vi "Read Fuel.vi"(8 "error in":errorcluster, 11 "Serial sessions":refnum<class "MB_Master_Serial.lvclass">[](array[class])) -> (0 "error out":errorcluster, 2 "Serial out":refnum<class "MB_Master_Serial.lvclass">[](array[class]), 3 "Fuel Flows":dbl[][](array[numeric]))   [LabVIEW 2017, in "Akwizycja.lvlib"]
uses:
  Akwizycja.lvlib
  <vilib>/Plasmionique/MB Master/MB_Master_Serial/MB_Master_Serial.lvclass
  D:/Program Files (x86)/National Instruments/LabVIEW 2017/vi.lib/Plasmionique/MB Master/MB_Master/MB_Master.lvclass
  <vilib>/Plasmionique/MB Master/MB Master.lvlib
  <vilib>/Utility/config.llb/NI_LVConfig.lvlib
panel:
  in  "P_Rx":T1
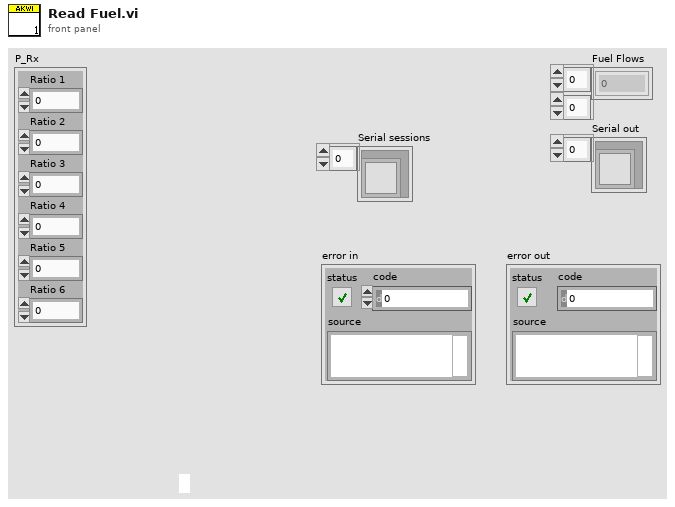
[diagram p1: front panel]
types:
  T1 = cluster{"Ratio 1":dbl, "Ratio 2":dbl, "Ratio 3":dbl, "Ratio 4":dbl, "Ratio 5":dbl, "Ratio 6":dbl}
  T2 = typedef "NI_LVConfig.lvlib/Config Data RefNum.ctl" = refnum<k1>
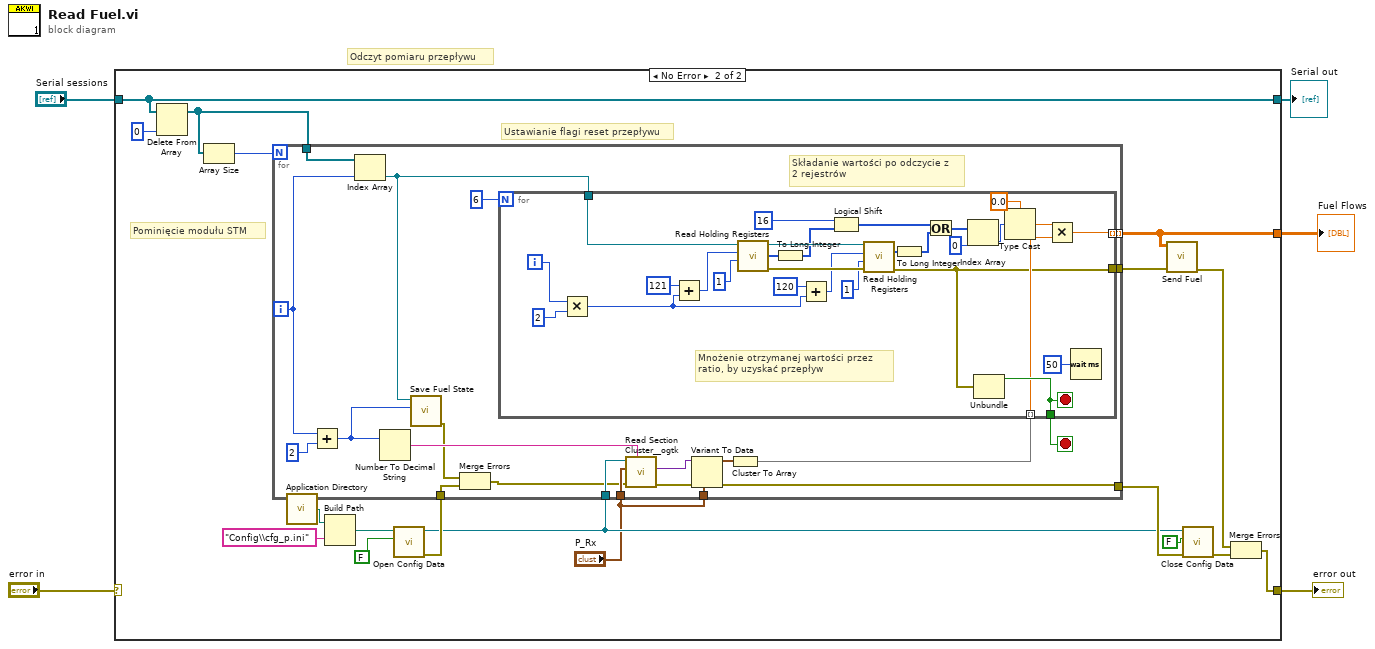
[diagram p0: block diagram]
diagram:
  # "Odczyt pomiaru przepływu"
  n1 = case shown="No Error" "error in" {
    selector: "error in" -> [w7 _]
    tunnel: "Serial sessions" -> [w6 w8]
    tunnel: [w7 w19] -> w4
    tunnel: [_ w10] -> w2
    tunnel: [w6 w8] -> w1
    frame Error {
    }
    frame No Error {
      # "Pominięcie modułu STM"
      # "Ustawianie flagi reset przepływu"
      n2 = Delete From Array(array=w8, index=0) -> (array with subset deleted=w9:refnum<class "MB_Master_Serial.lvclass">[])  [unwired: 1 in, 1 out]
      n3 = Array Size(array=w9) -> (size(s)=w16:i32)
      n4 = call <vilib>:"Application Directory.vi"() -> ("Application Directory"=w20:path)
      n5 = Build Path(base path=w20, name or relative path="Config\\cfg_p.ini") -> (appended path=w22:path)
      n6 = call <vilib>:"Open Config Data.vi"("create file if necessary (T)"=FALSE, "configuration file path"=w22) -> ("error out"=w18:errorcluster, "refnum"=w14:T2)  [unwired: 7 in, 1 out]
      n7 = for {
        N: w16 -> [_]
        tunnel: [w32] -> w25
        tunnel: w9 -> [w43]
        tunnel: [w45] -> w12
        tunnel: w18 -> [w28]
        tunnel: [w40] -> w10 mode=indexing
        tunnel: w14 -> [w39]
        tunnel: "P_Rx" -> [w38]
        tunnel: "P_Rx" -> [w35]
        i -> [w42]
        stop <- w44 stop-if-true
        # "Składanie wartości po odczycie z\n2 rejestrów"
        n8 = Add(x=w42, y=2) -> (x+y=w30:i32)
        n9 = Index Array(array=w43, index=w42) -> (element=w29:refnum<class "MB_Master_Serial.lvclass">)
        n10 = Number To Decimal String(number=w30) -> (decimal integer string=w37:string)  [unwired: 1 in]
        n11 = call "Save Fuel State.vi"("Slave ID"=w30, "Session in"=w29) -> ("error out"=w26:errorcluster)  [unwired: 9 in]
        n12 = Merge Errors(w26, w28) -> (w27:errorcluster)
        n13 = call <userlib>:"Read Section Cluster__ogtk.vi"("section (optional)"=w37, "error in (no error)"=w27, "Section Formatted Cluster Type"=w38, "refnum"=w39) -> ("error out"=w36:errorcluster, "Section Formatted Cluster"=w34:variant)  [unwired: 3 in, 3 out]
        n14 = Variant To Data(error in=w36, type=w35, Variant=w34) -> (data=w33:T1, error out=w32:errorcluster)
        n15 = Cluster To Array(cluster=w33) -> (array=w31:dbl[])
        n16 = for {
          N: 6 ("Numeric Control") -> [_]
          tunnel: w29 -> [w47]
          tunnel: [w48] -> w45
          tunnel: [w74] -> w44
          tunnel: [w55] -> w40 mode=indexing
          tunnel: w31 -> [w61] mode=indexing
          i -> [w66]
          stop <- w74 stop-if-true
          # "Mnożenie otrzymanej wartości przez \nratio, by uzyskać przepływ"
          n17 = Multiply(x=w66, y=2) -> (x*y=w64:i32)
          n18 = Add(x=u16 121 ("starting address"), y=w64) -> (x+y=w72:i32)
          n19 = call <vilib>:"Read Holding Registers.vi"("quantity"=u16 1, "starting address"=w72, "MB session in"=w47) -> ("error out"=w68:errorcluster, "Registers"=w54:u16[], "MB session out"=w69:refnum<class "MB_Master_Serial.lvclass">)  [unwired: 6 in]
          n20 = To Long Integer(number=w54) -> (32bit integer=w53:i32[])
          n21 = Add(x=u16 120 ("starting address"), y=w64) -> (x+y=w63:i32)
          n22 = Logical Shift(y=16, x=w53) -> (x << y=w58:i32[])
          n23 = call <vilib>:"Read Holding Registers.vi"("error in (no error)"=w68, "quantity"=u16 1, "starting address"=w63, "MB session in"=w69) -> ("error out"=w48:errorcluster, "Registers"=w59:u16[])  [unwired: 5 in, 1 out]
          n24 = To Long Integer(number=w59) -> (32bit integer=w60:i32[])
          n25 = Or(x=w58, y=w60) -> (x .or. y?=w57:i32[])
          n26 = Index Array(array=w57, index=0) -> (element=w52:i32)
          n27 = Unbundle(w48) -> ("status"=w74:bool)  [unwired: 2 out]
          n28 = Type Cast(type=sgl 0.0, x=w52) -> (*(type *) &x=w50:sgl)
          n29 = Multiply(x=w50, y=w61) -> (x*y=w55:dbl)
          n30 = Wait (ms)(milliseconds to wait=u32 50) -> ()  [unwired: 1 out]
        }
      }
      n31 = call "Send Fuel.vi"("error in"=w12, "Fuel Flows"=w10) -> ("error out"=w11:errorcluster)  [unwired: 9 in]
      n32 = call <vilib>:"Close Config Data.vi"("error in (no error)"=w25, "write file if changed (T)"=FALSE, "refnum"=w14) -> ("error out"=w17:errorcluster)  [unwired: 7 in, 1 out]
      n33 = Merge Errors(w11, w17) -> (w19:errorcluster)
    }
  }
  "error out" <- w4
  "Fuel Flows" <- w2
  "Serial out" <- w1
